vi "T-Periodic Triangle Gate.vi"(4 "Period T":dbl format="%#_4g", 9 "W":dbl format="%#_4g", 11 "t":dbl format="%#_4g") -> (3 "Triangle(t)":dbl format="%#_4g")   [LabVIEW 2019]
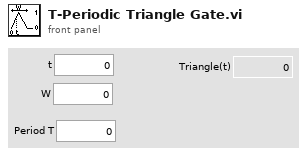
[diagram p1: front panel]
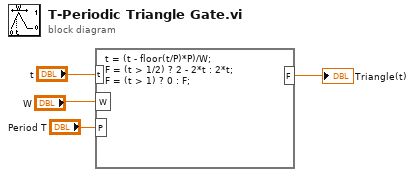
[diagram p0: block diagram]
diagram:
  n1 = formula code="t = (t - floor(t/P)*P)/W;\nF = (t > 1/2) ? 2 - 2*t : 2*t;\nF = (t > 1) ? 0 : F;"("t"="t", "W"="W", "P"="Period T") -> ("F"=→"Triangle(t)":dbl)
